vi "Apply and Save Changes.vi"(6 "Variant in":variant, 7 "Shift Pressed?":bool, 8 "error in (no error)":errorcluster, 10 "QD Combo Box Ref":refnum<vi>, 11 "QD Launch VI Ref":refnum<vi>) -> (0 "error out":errorcluster, 4 "Variant out":variant)   [LabVIEW 2024]
doc: "This shortcut helps to apply changes of the typedef and save the typedef.\n\nDefault Shortcut - [A]"
panel:
  in  "Undo Name":string="Quick Drop Keyboard Shortcut"
  # "Do not change the connector pane of this VI.\n\nSee the block diagram for directions on how to use this template."
  # "Specify the name of the Undo transaction"
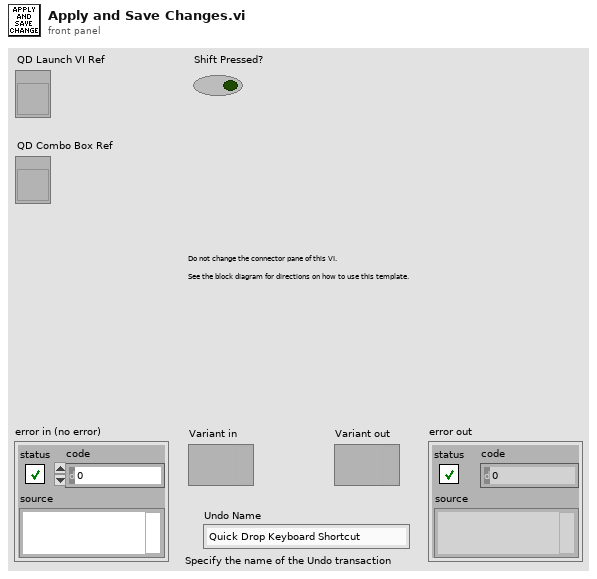
[diagram p1: front panel]
types:
  T1 = enum32{"invalid VI type", "Standard VI", "Control VI", "Global VI", "Polymorphic VI", "Configuration VI", "SubSystem", "Facade VI", "Method VI", "Statechart Diagram VI"}
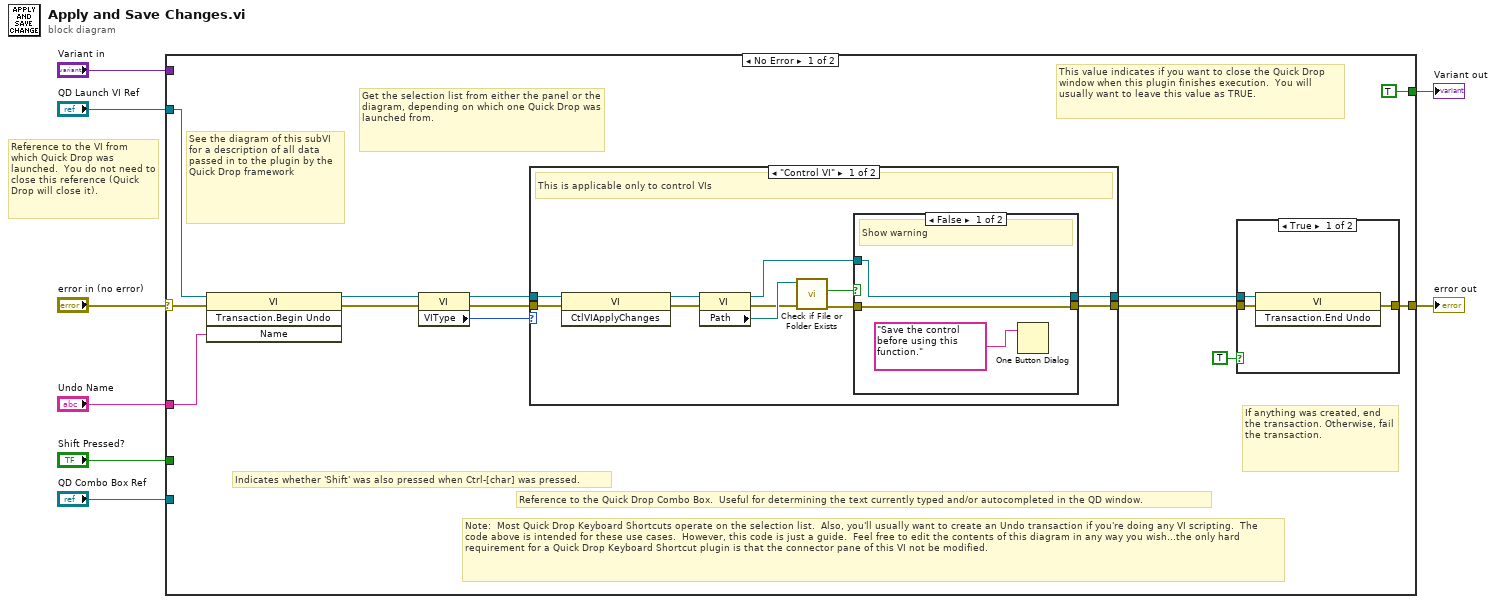
[diagram p0: block diagram]
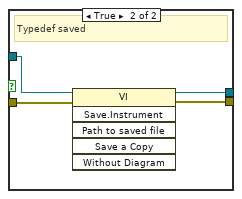
[diagram p2: hidden frame]
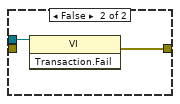
[diagram p4: hidden frame]
diagram:
  # "Reference to the VI from which Quick Drop was launched.  You do not need to close this reference (Quick Drop will close it)."
  n1 = case shown="No Error" "error in (no error)" {
    selector: "error in (no error)" -> [w21 w47]
    tunnel: [w17 w47] -> w7
    tunnel: "QD Launch VI Ref" -> [w20 _]
    tunnel: "Shift Pressed?" -> [_ _]
    tunnel: "QD Combo Box Ref" -> [_ _]
    tunnel: "Variant in" -> [_ _]
    tunnel: "Undo Name" -> [w19 _]
    tunnel: [TRUE _] -> w1
    frame No Error {
      # "Note:  Most Quick Drop Keyboard Shortcuts operate on the selection list.  Also, you'll usually want to create an Undo transaction if you're doing any VI scripting.  The code above is intended for these use cases.  However, this code is just a guide.  Feel free to edit the contents of this diagram in any way you wish...the only hard requirement for a Quick Drop Keyboard Shortcut plugin is that the connector pane of this VI not be modified."
      # "Get the selection list from either the panel or the diagram, depending on which one Quick Drop was launched from."
      # "If anything was created, end the transaction. Otherwise, fail the transaction."
      # "This value indicates if you want to close the Quick Drop window when this plugin finishes execution.  You will usually want to leave this value as TRUE."
      # "See the diagram of this subVI for a description of all data passed in to the plugin by the Quick Drop framework"
      # "Reference to the Quick Drop Combo Box.  Useful for determining the text currently typed and/or autocompleted in the QD window."
      # "Indicates whether 'Shift' was also pressed when Ctrl-[char] was pressed."
      n2 = invoke class="VI" method="Transaction.Begin Undo"(reference=w20, error in=w21, "Name"=w19) -> (reference out=w10:refnum<vi>, error out=w13:errorcluster)  [unwired: 1 in, 2 out]
      n3 = property class="VI"(reference=w10, error in=w13) -> (reference out=w15:refnum<vi>, error out=w14:errorcluster, "VIType"=w16:T1)
      n4 = case shown="\"Control VI\"" w16 {
        tunnel: w15 -> [w30 w40]
        tunnel: w14 -> [w29 w41]
        tunnel: [w32 w41] -> w12
        tunnel: [w31 w40] -> w9
        frame "Control VI" {
          # "This is applicable only to control VIs"
          n5 = invoke class="VI" method="CtlVIApplyChanges"(reference=w30, error in=w29) -> (reference out=w28:refnum<vi>, error out=w27:errorcluster)  [unwired: 1 in, 1 out]
          n6 = property class="VI"(reference=w28, error in=w27) -> (reference out=w22:refnum<vi>, error out=w25:errorcluster, "Path"=w26:path)
          n7 = call <vilib>:"Check if File or Folder Exists.vi"("error in (no error)"=w25, "path"=w26) -> ("error out"=w24:errorcluster, "file or folder exists?"=w23:bool)  [unwired: 7 in, 1 out]
          n8 = case shown="False" w23 {
            tunnel: [w35 w39] -> w32
            tunnel: [w34 w38] -> w31
            tunnel: w24 -> [w35 w37]
            tunnel: w22 -> [w34 w36]
            frame False {
              # "Show warning"
              n9 = One Button Dialog(message="Save the control before using this function.") -> ()  [unwired: 1 in, 1 out]
            }
            frame True {
              # "Typedef saved"
              n10 = invoke class="VI" method="Save.Instrument"(reference=w36, error in=w37) -> (reference out=w38:refnum<vi>, error out=w39:errorcluster)  [unwired: 4 in, 4 out]
            }
          }
        }
        frame Default {
        }
      }
      n11 = case shown="True" TRUE {
        tunnel: w9 -> [w43 w45]
        tunnel: [w44 w46] -> w17
        tunnel: w12 -> [w42 _]
        frame True {
          n12 = invoke class="VI" method="Transaction.End Undo"(reference=w43, error in=w42) -> (error out=w44:errorcluster)  [unwired: 1 in, 2 out]
        }
        frame False {
          n13 = invoke class="VI" method="Transaction.Fail"(reference=w45) -> (error out=w46:errorcluster)  [unwired: 2 in, 2 out]
        }
      }
    }
    frame Error {
    }
  }
  "error out" <- w7
  "Variant out" <- w1
